vi "Add Child.vi"(4 "Position":i32[](array[numeric]), 6 "Tree Item In":T1, 8 "error in (no error)":errorcluster, 9 "Data In":refnum<class "Tree Data.lvclass">, 10 "Tree In":refnum<class "Tree.lvclass">, 11 "Composite Tree Data in":refnum<class "Composite Tree Data.lvclass">) -> (0 "error out":errorcluster, 2 "Tree Out":refnum<class "Tree.lvclass">, 3 "Composite Tree Data out":refnum<class "Composite Tree Data.lvclass">)   [LabVIEW 2019, in "Composite Tree Data.lvclass"]
uses:
  Composite Tree Data.lvclass
  C:/Users/iio/Desktop/NTHU Brain Center/General Purpose/Classes/Ancestor/Front Panel Container/Tree/Tree Data/Tree Data.lvclass
  Tree Data/Tree Data.lvclass
  Tree/Tree.lvclass
  Tree/Type Def/Tree Item.ctl
  Composite Tree Data.lvclass/Composite Tree Data.ctl
  Tree Data/Tree Data.lvclass/Tree Data.ctl
  Tree/Tree.lvclass/Tree.ctl
  Tree/Public Data/Read Root Tag.vi
  Tree Data/Protected Data/Read Tag.vi
  Polymorphic VIs/Tree Converter/Tag To BFS Index.vi
  Polymorphic VIs/Tree Converter/BFS Index To Tag.vi
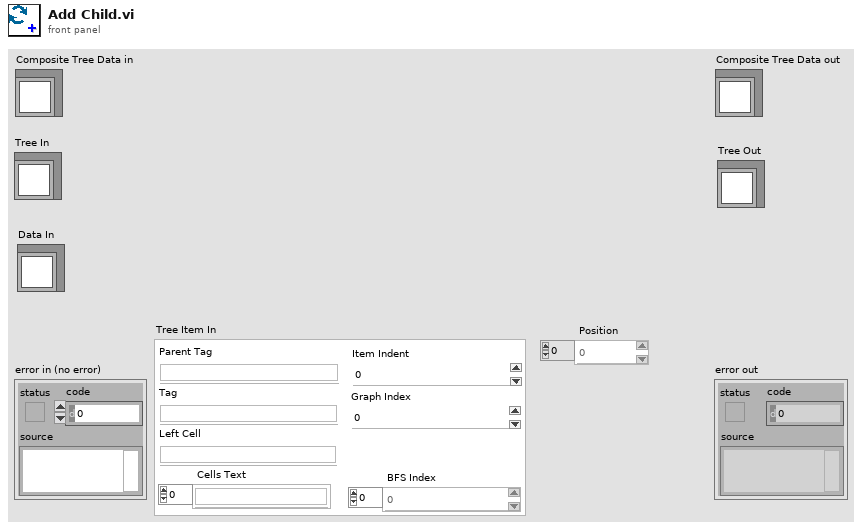
[diagram p1: front panel]
types:
  T1 = typedef "Tree Item.ctl" = cluster{"Parent Tag":string, "Tag":string, "Left Cell":string, "Cells Text":string[], "BFS Index":i32[], "Graph Index":i32, "Item Indent":i32}
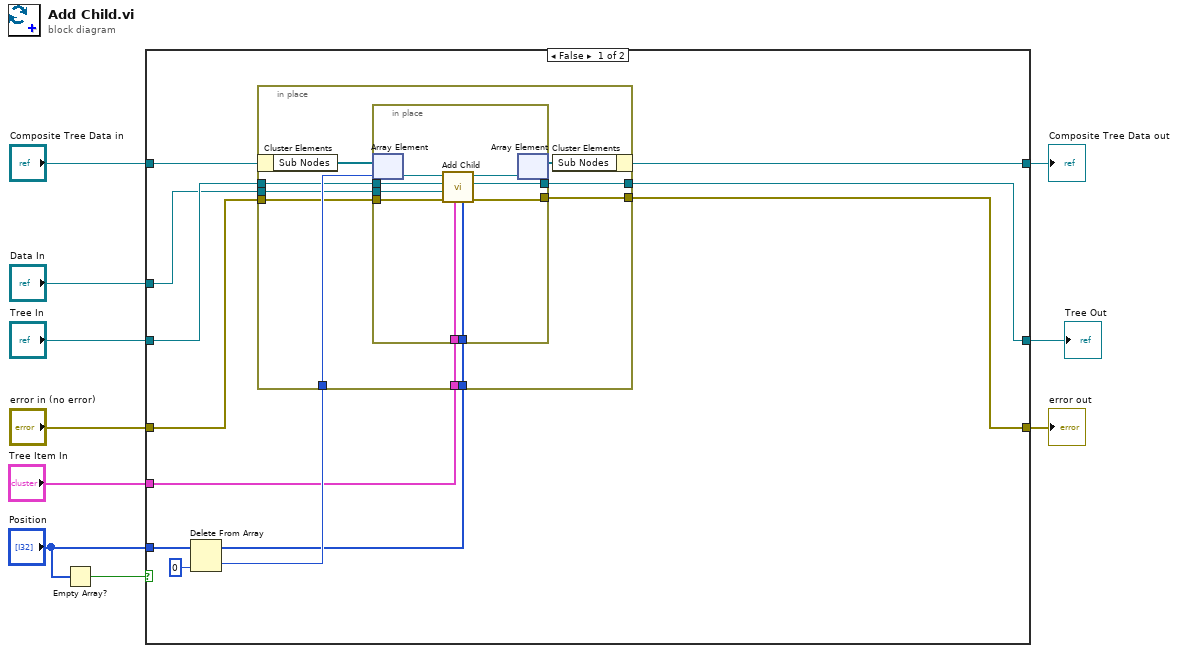
[diagram p0: block diagram]
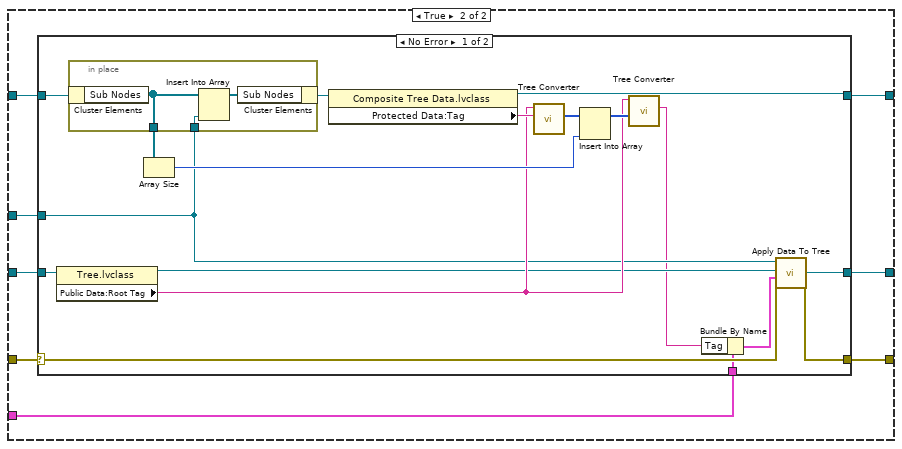
[diagram p2: hidden frame]
diagram:
  n1 = Empty Array?(array="Position") -> (empty?=w2:bool)
  n2 = case shown="False" w2 {
    tunnel: "error in (no error)" -> [w15 w49]
    tunnel: [w14 w48] -> w9
    tunnel: "Composite Tree Data in" -> [w20 w47]
    tunnel: [w19 w46] -> w7
    tunnel: "Data In" -> [w13 w45]
    tunnel: [w16 w44] -> w5
    tunnel: "Tree In" -> [w17 w43]
    tunnel: "Tree Item In" -> [w12 w42]
    tunnel: "Position" -> [w22 _]
    frame False {
      n3 = Delete From Array(array=w22, index=0) -> (deleted portion=w18:i32, array with subset deleted=w11:i32[])  [unwired: 1 in]
      n4 = in-place {
        in-place-border: w18 -> [w31]
        in-place-border: w17 -> [w29]
        in-place-border: [w28] -> w16
        in-place-border: w15 -> [w27]
        in-place-border: [w26] -> w14
        in-place-border: w13 -> [w25]
        in-place-border: w12 -> [w24]
        in-place-border: w11 -> [w23]
        n5 = in-place-cluster #1(w20) -> ("Sub Nodes"=w32:refnum<class "Tree Data.lvclass">[])
        n6 = in-place {
          in-place-border: w29 -> [w39]
          in-place-border: [w38] -> w28
          in-place-border: w27 -> [w37]
          in-place-border: [w36] -> w26
          in-place-border: w25 -> [w35]
          in-place-border: w24 -> [w34]
          in-place-border: w23 -> [w33]
          n7 = in-place-array #2(w32, w31) -> (w41:refnum<class "Tree Data.lvclass">)
          n8 = call-dynamic "Add Child.vi"("Position"=w33, "Tree Item In"=w34, "error in (no error)"=w37, "Data In"=w35, "Tree In"=w39, "Tree Data in"=w41) -> ("error out"=w36:errorcluster, "Tree Out"=w38:refnum<class "Tree.lvclass">, "Tree Data out"=w40:refnum<class "Tree Data.lvclass">)  [unwired: 3 in]
          n9 = in-place-array #2(w40) -> (w30:refnum<class "Tree Data.lvclass">[])  [unwired: 1 out]
        }
        n10 = in-place-cluster #1("Sub Nodes"=w30) -> (w19:refnum<class "Composite Tree Data.lvclass">)
      }
    }
    frame True {
      n11 = case shown="No Error" w49 {
        selector: w49 -> [w56 w73]
        tunnel: [w53 w73] -> w48
        tunnel: [w65 w72] -> w46
        tunnel: w47 -> [w67 w72]
        tunnel: w45 -> [w54 _]
        tunnel: [w57 w71] -> w44
        tunnel: w43 -> [w64 w71]
        tunnel: w42 -> [w52 _]
        frame No Error {
          n12 = property class="Tree.lvclass"(reference=w64) -> (reference out=w55:refnum<class "Tree.lvclass">, "Public Data:Root Tag"=w58:string)  [unwired: 1 in, 1 out]
          n13 = in-place {
            in-place-border: w54 -> [w69]
            in-place-border: [w68] -> w62
            n14 = in-place-cluster #3(w67) -> ("Sub Nodes"=w68:refnum<class "Tree Data.lvclass">[])
            n15 = Insert Into Array(array=w68, new element=w69) -> (w70:refnum<class "Tree Data.lvclass">[])  [unwired: 1 in]
            n16 = in-place-cluster #3("Sub Nodes"=w70) -> (w66:refnum<class "Composite Tree Data.lvclass">)
          }
          n17 = Array Size(array=w62) -> (size(s)=w60:i32)
          n18 = property class="Composite Tree Data.lvclass"(reference=w66) -> (reference out=w65:refnum<class "Composite Tree Data.lvclass">, "Protected Data:Tag"=w63:string)  [unwired: 1 in, 1 out]
          n19 = call-poly "Tree Converter.vi"("Tag In"=w63, "Root Tag"=w58) -> ("BFS Index Out"=w61:i32[])  [unwired: 9 in]
          n20 = Insert Into Array(array=w61, new element=w60) -> (w59:i32[])  [unwired: 1 in]
          n21 = call-poly "Tree Converter.vi"("BFS Index In"=w59, "Root Tag In"=w58) -> ("Tag Out"=w51:string)  [unwired: 9 in]
          n22 = Bundle By Name(cluster=w52, "Tag"=w51) -> (w50:T1)
          n23 = call-dynamic "Apply Data To Tree.vi"("error in (no error)"=w56, "Tree Item In"=w50, "Tree In"=w55, "Tree Data in"=w54) -> ("error out"=w53:errorcluster, "Tree Out"=w57:refnum<class "Tree.lvclass">)  [unwired: 5 in, 1 out]
        }
        frame Error {
        }
      }
    }
  }
  "error out" <- w9
  "Composite Tree Data out" <- w7
  "Tree Out" <- w5
